vi "Vision Center RPM Shoot.vi"(0 "Intake":dbl=1.0, 1 "X axis value":dbl=0.05 format="%#_13g", 2 "X axis value 2":dbl=-0.05, 3 "Distance Type":enum16{"SONAR", "VISION", "BOTH"}(ring)=enum."VISION") -> ()   [LabVIEW 2015]
uses:
  Robot Global Data.vi
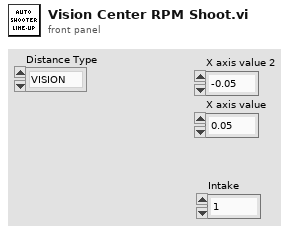
[diagram p1: front panel]
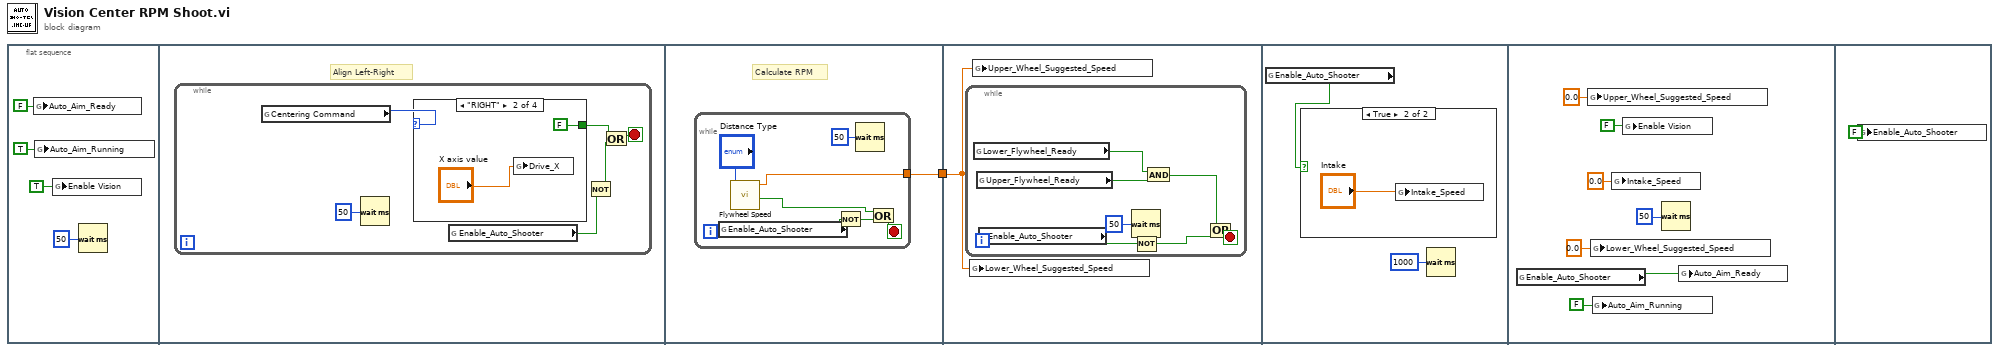
[diagram p0: block diagram]
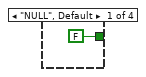
[diagram p2: hidden frame]
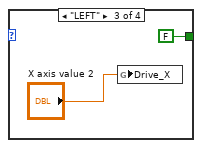
[diagram p3: hidden frame]
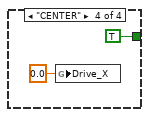
[diagram p4: hidden frame]
diagram:
  n1 = flat-sequence {
    tunnel: [w19] -> w1
    tunnel: w1 -> [w27]
    frame #0 {
      n2 = global write "Robot Global Data.vi" "Auto_Aim_Ready"(FALSE ("Auto_Aim_Ready")) -> ()
      n3 = global write "Robot Global Data.vi" "Auto_Aim_Running"(TRUE ("Auto_Aim_Running")) -> ()
      n4 = global write "Robot Global Data.vi" "Enable Vision"(TRUE ("Enable Vision")) -> ()
      n5 = Wait (ms)(milliseconds to wait=u32 50) -> ()  [unwired: 1 out]
    }
    frame #1 {
      # "Align Left-Right"
      n6 = while {
        stop <- w8 stop-if-true
        n7 = global read "Robot Global Data.vi" "Centering Command"() -> (w10:enum16{"NULL", "RIGHT", "LEFT", "CENTER"})
        n8 = Wait (ms)(milliseconds to wait=u32 50) -> ()  [unwired: 1 out]
        n9 = case shown="\"RIGHT\"" w10 {
          tunnel: [FALSE FALSE FALSE TRUE] -> w11
          frame "NULL", Default {
          }
          frame "RIGHT" {
            n10 = global write "Robot Global Data.vi" "Drive_X"("X axis value") -> ()
          }
          frame "LEFT" {
            n11 = global write "Robot Global Data.vi" "Drive_X"("X axis value 2") -> ()
          }
          frame "CENTER" {
            n12 = global write "Robot Global Data.vi" "Drive_X"(0.0 ("Drive_X")) -> ()
          }
        }
        n13 = global read "Robot Global Data.vi" "Enable_Auto_Shooter"() -> (w7:bool)
        n14 = Not(x=w7) -> (.not. x?=w6:bool)
        n15 = Or(x=w11, y=w6) -> (x .or. y?=w8:bool)
      }
    }
    frame #2 {
      # "Calculate RPM"
      n16 = while {
        tunnel: [w26] -> w19
        stop <- w23 stop-if-true
        n17 = global read "Robot Global Data.vi" "Enable_Auto_Shooter"() -> (w22:bool)
        n18 = call "Flywheel Speed.vi"("Distance Type"="Distance Type") -> ("Calculation_Ready"=w20:bool, "Suggested Speed"=w26:dbl)  [unwired: 8 in, 1 out]
        n19 = Not(x=w22) -> (.not. x?=w21:bool)
        n20 = Wait (ms)(milliseconds to wait=u32 50) -> ()  [unwired: 1 out]
        n21 = Or(x=w20, y=w21) -> (x .or. y?=w23:bool)
      }
    }
    frame #3 {
      n22 = while {
        stop <- w30 stop-if-true
        n23 = global read "Robot Global Data.vi" "Lower_Flywheel_Ready"() -> (w33:bool)
        n24 = global read "Robot Global Data.vi" "Upper_Flywheel_Ready"() -> (w34:bool)
        n25 = global read "Robot Global Data.vi" "Enable_Auto_Shooter"() -> (w29:bool)
        n26 = Wait (ms)(milliseconds to wait=u32 50) -> ()  [unwired: 1 out]
        n27 = Not(x=w29) -> (.not. x?=w28:bool)
        n28 = And(x=w33, y=w34) -> (x .and. y?=w32:bool)
        n29 = Or(x=w32, y=w28) -> (x .or. y?=w30:bool)
      }
      n30 = global write "Robot Global Data.vi" "Lower_Wheel_Suggested_Speed"(w27) -> ()
      n31 = global write "Robot Global Data.vi" "Upper_Wheel_Suggested_Speed"(w27) -> ()
    }
    frame #4 {
      n32 = global read "Robot Global Data.vi" "Enable_Auto_Shooter"() -> (w35:bool)
      n33 = case shown="True" w35 {
        frame False {
        }
        frame True {
          n34 = global write "Robot Global Data.vi" "Intake_Speed"("Intake") -> ()
        }
      }
      n35 = Wait (ms)(milliseconds to wait=u32 1000) -> ()  [unwired: 1 out]
    }
    frame #5 {
      n36 = global read "Robot Global Data.vi" "Enable_Auto_Shooter"() -> (w38:bool)
      n37 = global write "Robot Global Data.vi" "Upper_Wheel_Suggested_Speed"(0.0 ("Upper_Wheel_Suggested_Speed")) -> ()
      n38 = global write "Robot Global Data.vi" "Lower_Wheel_Suggested_Speed"(0.0 ("Lower_Wheel_Suggested_Speed")) -> ()
      n39 = global write "Robot Global Data.vi" "Auto_Aim_Running"(FALSE ("Auto_Aim_Running")) -> ()
      n40 = global write "Robot Global Data.vi" "Intake_Speed"(0.0 ("Intake_Speed")) -> ()
      n41 = global write "Robot Global Data.vi" "Enable Vision"(FALSE ("Enable Vision")) -> ()
      n42 = Wait (ms)(milliseconds to wait=u32 50) -> ()  [unwired: 1 out]
      n43 = global write "Robot Global Data.vi" "Auto_Aim_Ready"(w38) -> ()
    }
    frame #6 {
      n44 = global write "Robot Global Data.vi" "Enable_Auto_Shooter"(FALSE ("Enable_Shooter")) -> ()
    }
  }
